vi "保存表格列首设定.vi"() -> (1 "复锁拍螺帽":string[](array[string])=["批次号", "拍照时间", "结果", "PCB序号", "单片PCB点位序号", "螺帽中心X", "螺帽中心Y", "一字槽角度", "螺帽内径", "一字槽两边角度差异", "一字槽宽度", "视觉补偿量X", "视觉补偿量Y", "螺丝刀要旋转角度", "取料点相对拍照点偏移X", "取料点相对拍照点偏移Y", "取料点Z", "取料点R", "拧紧程式序号1", "拧紧程式序号2", "", "", "", ""], 2 "取料拍螺帽":string[](array[string])=["批次号", "拍照时间", "结果", "PCB序号", "单片PCB点位序号", "螺帽中心X", "螺帽中心Y", "一字槽角度", "螺帽内径", "一字槽两边角度差异", "一字槽宽度", "视觉补偿量X", "视觉补偿量Y", "螺丝刀要旋转角度", "取料点相对拍照点偏移X", "取料点相对拍照点偏移Y", "取料点Z", "取料点R", "拧紧程式序号1", "拧紧程式序号2", "放料点坐标-X", "放料点坐标-Y", "放料点坐标-Z", "放料点坐标-R"], 3 "拍PCB孔信息":string[](array[string])=["批次号", "拍照时间", "结果", "PCB序号", "单片PCB点位序号", "孔中心坐标X", "孔中心坐标Y", "孔半径", "视觉补偿值X", "视觉补偿值Y"])   [LabVIEW 2014]
panel:
  out "数组":string[](array[string])
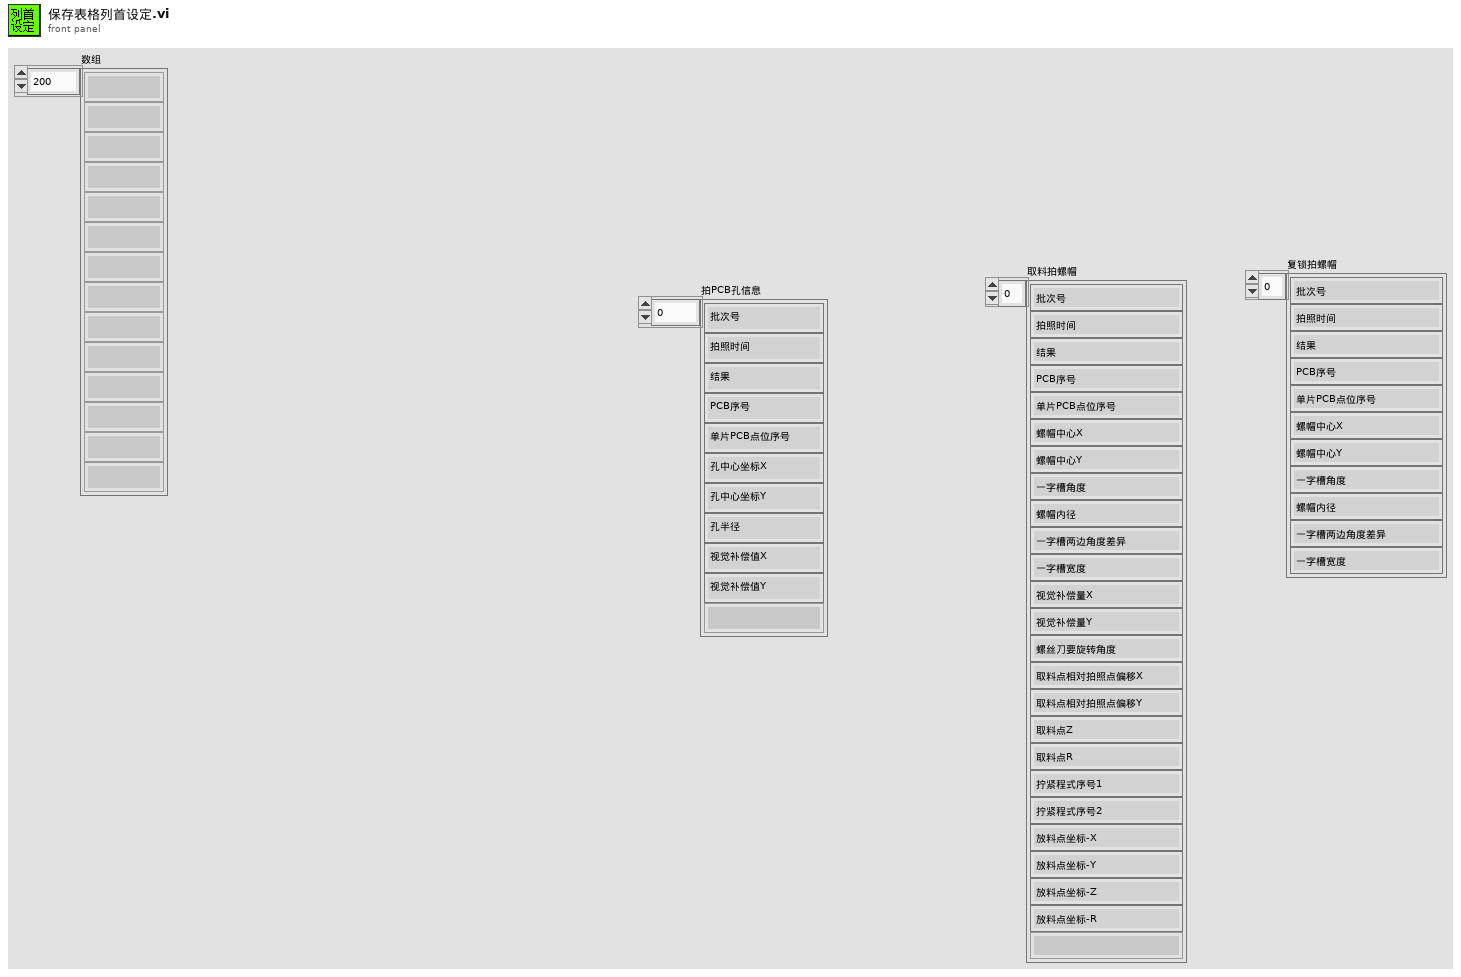
[diagram p1: front panel]
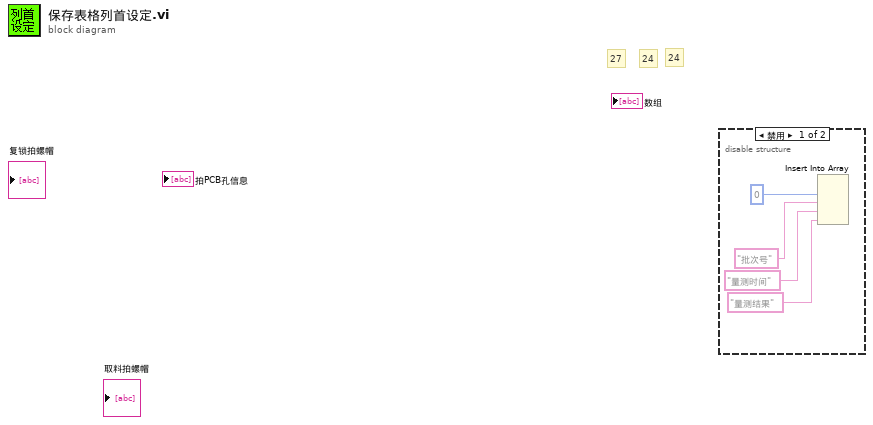
[diagram p0: block diagram]
diagram:
  # "27"
  # "24"
  # "24"
  n1 = disable-structure shown="禁用" {
    frame Disabled {
      n2 = Insert Into Array(index=0 ("索引"), new element #1="批次号" ("新元素/子数组"), new element #2="量测时间" ("新元素/子数组"), new element #3="量测结果" ("新元素/子数组")) -> ()  [unwired: 1 in, 1 out]
    }
    frame Enabled {
    }
  }
